vi "Submit.vi"(0 "NI Build Specification_LV In":refnum<class "NI Build Specification_LV.lvclass">) -> (4 "NI Build Specification_LV Out":refnum<class "NI Build Specification_LV.lvclass">)   [LabVIEW 2017, in "CL_G3_VIComponentBuilder.lvlib" / "NI Build Specification_LV.lvclass"]
doc: "Invokes the commit behaivor specified by this export and any additional operations deemed necessary by the export. \n <MustCallParent>The parent overwrites the original LabVIEW Project with the exported LabVIEW Project and therefore must be called from any child.</MustCallParent>"
uses:
  NI Build Specification_LV.lvclass
  C:/Tool Chain Support/Software Module Builder/Source/Exports/Exports/Export.lvclass
  Exports/Export.lvclass/Export.ctl
  Exports/Accessors/Write Export Operation Errors.vi
  Exports/Accessors/Read Commit behavior.vi
  Exports/Accessors/Read Exported Build Specification Path.vi
  Exports/Accessors/Read Export Build Specification.vi
  Exports/Accessors/Read Export Operation Errors.vi
  Commit Behavior/Commit/Commit.lvclass
  Exports/Export.lvclass
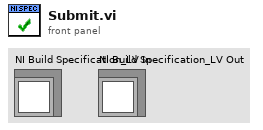
[diagram p1: front panel]
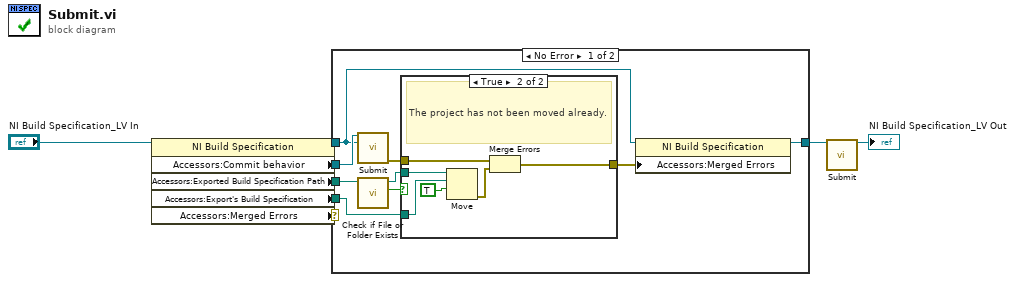
[diagram p0: block diagram]
diagram:
  n1 = property class="NI Build Specification"(reference="NI Build Specification_LV In") -> (reference out=w6:refnum<class "NI Build Specification_LV.lvclass">, "Accessors:Commit behavior"=w7:refnum<class "Commit.lvclass">, "Accessors:Exported Build Specification Path"=w4:path, "Accessors:Export's Build Specification"=w5:path, "Accessors:Merged Errors"=w1:errorcluster)  [unwired: 1 in, 1 out]
  n2 = case shown="No Error" w1 {
    tunnel: w7 -> [w17 _]
    tunnel: w6 -> [w16 w25]
    tunnel: w5 -> [w15 _]
    tunnel: w4 -> [w12 _]
    tunnel: [w9 w25] -> w2
    frame No Error {
      n3 = call-dynamic "Submit.vi"("Commit in"=w17, "Export"=w16) -> ("error out"=w14:errorcluster)  [unwired: 12 in, 1 out]
      n4 = call <vilib>:"Check if File or Folder Exists.vi"("path"=w12) -> ("file or folder exists?"=w10:bool, "dup path"=w11:path)  [unwired: 8 in, 1 out]
      n5 = case shown="True" w10 {
        tunnel: w15 -> [_ w23]
        tunnel: w14 -> [w18 w22]
        tunnel: [w18 w20] -> w13
        tunnel: w11 -> [_ w19]
        frame False {
          # "The project was already moved as a result of the the project owning multiple exports."
        }
        frame True {
          # "The project has not been moved already."
          n6 = Move(source path=w19, 9:TRUE ("overwrite (F)"), 10:w23) -> (error out=w21:errorcluster)  [unwired: 2 in, 2 out]
          n7 = Merge Errors(w22, w21) -> (w20:errorcluster)
        }
      }
      n8 = property class="NI Build Specification"(reference=w16, "Accessors:Merged Errors"=w13) -> (reference out=w9:refnum<class "NI Build Specification_LV.lvclass">)  [unwired: 1 in, 1 out]
    }
    frame Error {
    }
  }
  n9 = call-parent "Submit.vi"("Export In"=w2) -> ("Export Out"=→"NI Build Specification_LV Out":refnum<class "NI Build Specification_LV.lvclass">)  [unwired: 14 in]
